vi "command add sync in action calb.vi"(8 "error in (no error)":errorcluster, 9 "calibration":cluster{"A":dbl, "MicrostepMode":u32}, 10 "the_command_add_sync_in_action_calb":cluster{"Position":sgl, "Time":u32}, 11 "id":i32) -> (0 "error out":errorcluster, 3 "function return":i32)   [LabVIEW 2012, in "libximc.lvlib"]
doc: "result_t XIMC_API command_add_sync_in_action_calb (device_t id, const command_add_sync_in_action_calb_t* the_command_add_sync_in_action_calb, const calibration_t* calibration);"
uses:
  libximc.lvlib
  libximc.dll
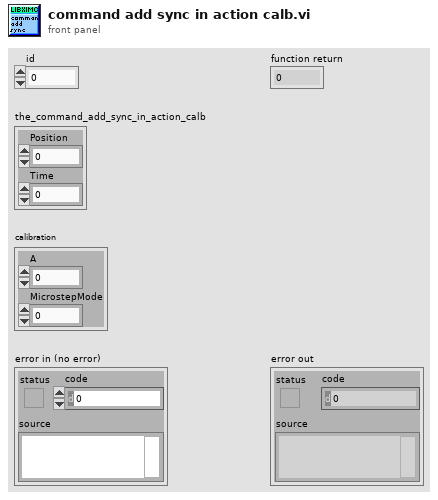
[diagram p1: front panel]
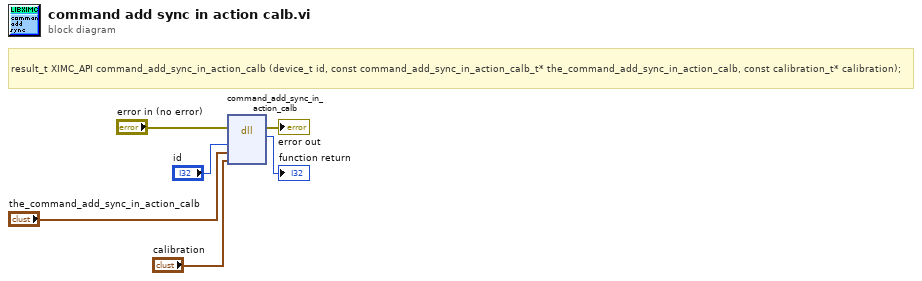
[diagram p0: block diagram]
diagram:
  # "result_t XIMC_API command_add_sync_in_action_calb (device_t id, const command_add_sync_in_action_calb_t* the_command_add_sync_in_action_calb, const calibration_t* calibration);"
  n1 = dll-call lib="E:/labview-2.12.1-Labview_12.0/ximcLVx32/libximc.*" fn="command_add_sync_in_action_calb"(error in="error in (no error)", "id"="id", "the_command_add_sync_in_action_calb"="the_command_add_sync_in_action_calb", "calibration"="calibration") -> (error out=→"error out":errorcluster, →"function return":i32)  [unwired: 5 in, 1 out]
